vi "日志报警状态存储 (子VI).vi"() -> ()   [LabVIEW 2016, in "斯坦道CODMn.lvlib"]
uses:
  <vilib>/ptbypt/NI_PtbyPt.lvlib
panel:
  out "多列列表框":i32(listbox)
  out "CODMn工作状态":T1(ring)
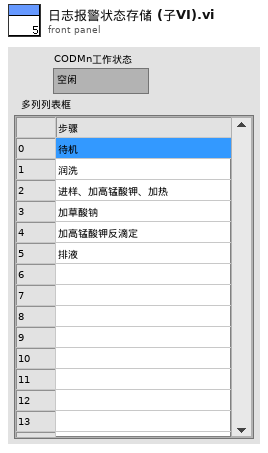
[diagram p1: front panel]
types:
  T1 = enum16{"空闲", "水样测试", "标样核查", "零点核查", "跨度核查", "空白测试", "平行样测试", "质控样", "空白校准", "标样校准", "加标回收"}
  T2 = cluster{"时间标识":timestamp, "设备":string, "日志信息":string, "备注":string}
  T3 = cluster{"时间标识":timestamp, "参数":string, "日志信息":string, "流程参数":string}
  T4 = cluster{"ORP故障":bool, "温控器故障":bool, "加热故障":bool, "高锰酸钾报警":bool, "草酸钠报警":bool, "测量错误":bool, "校零错误":bool, "校标错误":bool, " 进水样超量程":bool, "排液阀故障":bool, "60分钟超时报警":bool, "进样无液体报警":bool}
  T5 = typedef "数据库类型.ctl" = enum16{"Access", "SQLite"}
  T6 = cluster{"测量量程":dbl, "测量精度":dbl, "测量间隔":dbl, "消解温度":dbl, "消解时长":dbl, "空白校准时间":timestamp, "曲线截距":dbl, "曲线斜率":dbl, "测量检出限":dbl, "测量信号值":dbl, "线性相关系数":dbl, "二次多项式系数":dbl, "标样校准时间":timestamp, "稀释倍数":dbl, "三项式系数":dbl, "空白标定系数":dbl, "量程系数":dbl, "F0/ORPA":dbl, "F1/ORPB":dbl, "F2/ORPK":dbl, "F3":dbl, "F4":dbl, "F5":dbl, "F6":dbl, "F7":dbl, "X0/滴定数":dbl, "量程":dbl}
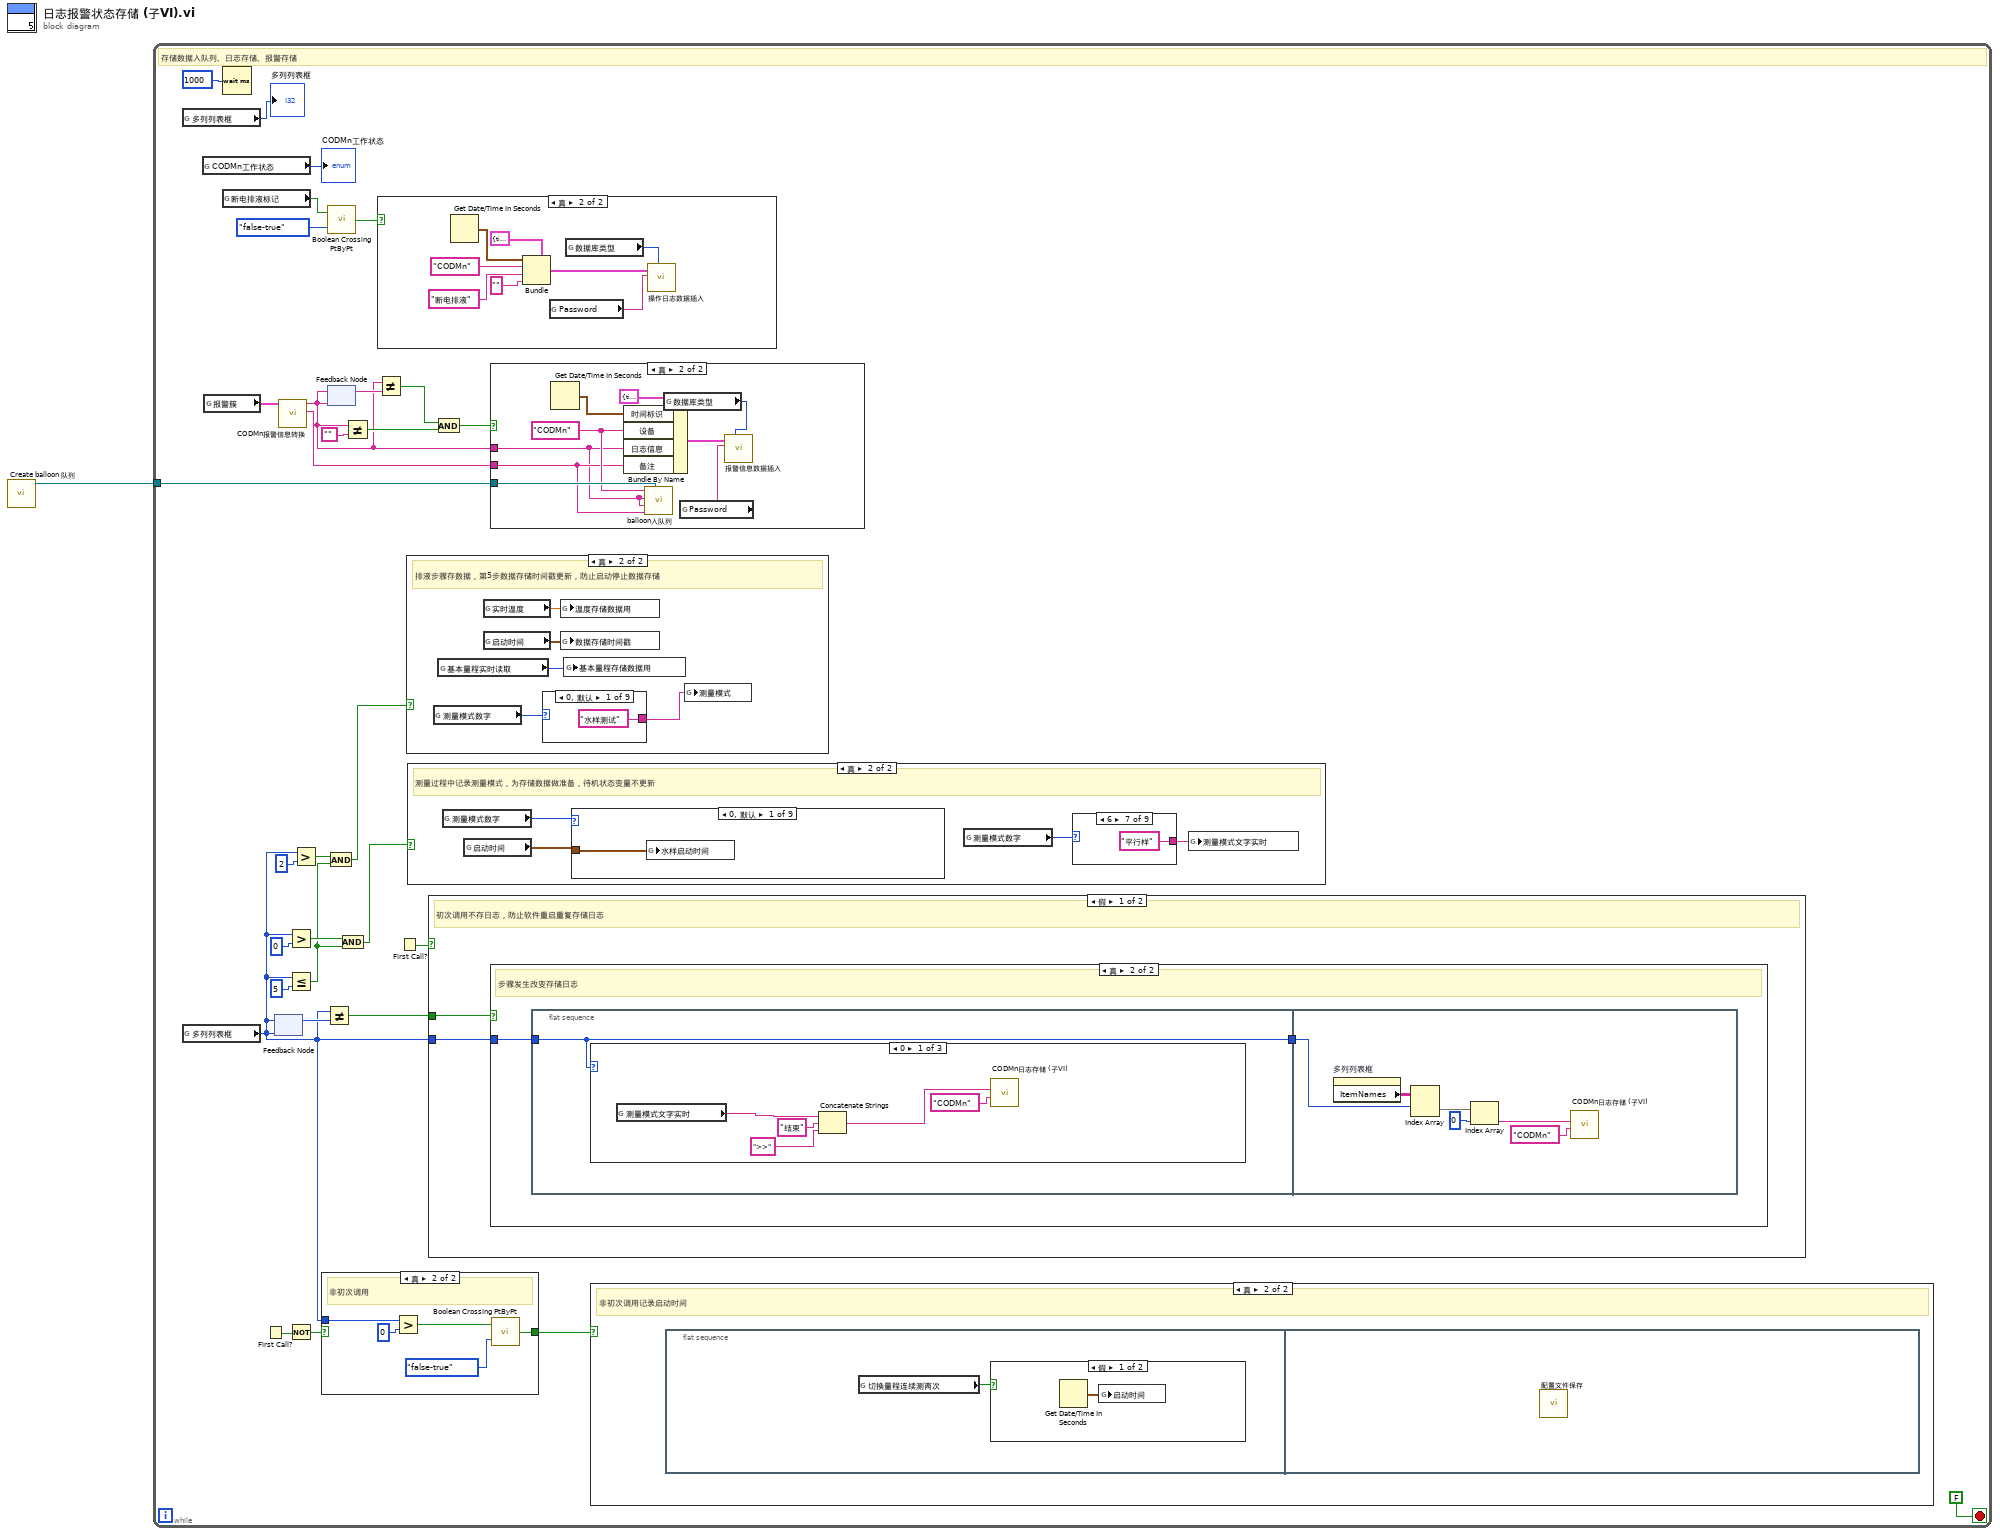
[diagram p0: block diagram]
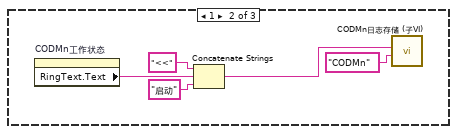
[diagram p3: hidden frame]
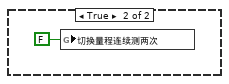
[diagram p10: hidden frame]
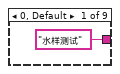
[diagram p12: hidden frame]
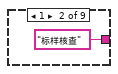
[diagram p13: hidden frame]
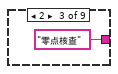
[diagram p14: hidden frame]
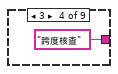
[diagram p15: hidden frame]
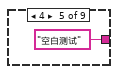
[diagram p16: hidden frame]
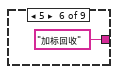
[diagram p17: hidden frame]
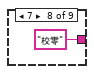
[diagram p18: hidden frame]
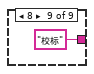
[diagram p19: hidden frame]
diagram:
  n1 = call "Create balloon 队列.vi"() -> ("队列输出"=w1:refnum<queue>)  [unwired: 11 in]
  n2 = while {
    tunnel: w1 -> [w2]
    stop <- FALSE stop-if-true
    # "存储数据入队列、日志存储、报警存储"
    n3 = global read "运行时序全局变量.vi" "多列列表框"() -> (→"多列列表框":i32)
    n4 = global read "运行时序全局变量.vi" "多列列表框"() -> (w6:i32)
    n5 = global read "COD测量模式全局.vi" "CODMn工作状态"() -> (→"CODMn工作状态":T1)
    n6 = global read "COD内部交互全局.vi" "报警簇"() -> (w13:T4)
    n7 = global read "COD内部交互全局.vi" "断电排液标记"() -> (w12:bool)
    n8 = Wait (ms)(milliseconds to wait=u32 1000 ("等待时间（毫秒）")) -> ()  [unwired: 1 out]
    n9 = First Call?() -> (First Call?: T/F=w16:bool)
    n10 = feedback #1(w6) -> (w27:i32)
    n11 = feedback-in #1(w6) -> ()
    n12 = call "CODMn报警信息转换.vi"("报警簇"=w13) -> ("CODMN报警信息备注"=w3:string, "CODMN报警信息"=w17:string)  [unwired: 9 in]
    n13 = Greater?(x=w6, y=u16 0) -> (0:w32:bool)
    n14 = Less Or Equal?(x=w6, y=u16 5) -> (x <= y?=w7:bool)
    n15 = Not(x=w16) -> (.not. x?=w14:bool)
    n16 = Greater?(x=w6, y=u16 2) -> (0:w8:bool)
    n17 = case shown="真" w14 {
      selector: w14 -> [w54 _]
      tunnel: w6 -> [_ w56]
      tunnel: [w54 w55] -> w15
      frame False {
      }
      frame True {
        # "非初次调用"
        n18 = Greater?(x=w56, y=u16 0) -> (0:w59:bool)
        n19 = call <vilib>:"Boolean Crossing PtByPt.vi"("direction"=enum16{"either", "false-true", "true-false"}."false-true", "input"=w59) -> ("crossing"=w55:bool)  [unwired: 1 in]
      }
    }
    n20 = Not Equal?(x=w6, y=w27) -> (x != y?=w28:bool)
    n21 = call <vilib>:"Boolean Crossing PtByPt.vi"("direction"=enum16{"either", "false-true", "true-false"}."false-true", "input"=w12) -> ("crossing"=w23:bool)  [unwired: 1 in]
    n22 = feedback #2(w17) -> (w18:string)
    n23 = feedback-in #2(w17) -> ()
    n24 = And(x=w8, y=w7) -> (x .and. y?=w5:bool)
    n25 = And(x=w32, y=w7) -> (x .and. y?=w4:bool)
    n26 = Not Equal?(x=w17, y="") -> (x != y?=w22:bool)
    n27 = Not Equal?(x=w17, y=w18) -> (x != y?=w19:bool)
    n28 = case shown="真" w23 {
      frame False {
      }
      frame True {
        n29 = Get Date/Time In Seconds() -> (seconds since 1Jan1904=w76:timestamp)
        n30 = Bundle(cluster=T3 {"时间标识"=timestamp(0 s since 1904-01-01), "参数"="", "日志信息"="", "流程参数"=""} ("data in"), "时间标识"=w76, "参数"="CODMn" ("table输入"), "日志信息"="断电排液", "流程参数"="" ("table输入")) -> (w71:T3)
        n31 = global read "CODMn断电保存全局变量.vi" "Password"() -> (w69:string)
        n32 = global read "CODMn断电保存全局变量.vi" "数据库类型"() -> (w70:T5)
        n33 = call "操作日志数据插入.vi"("data"=w71, "Password"=w69, "数据库类型"=w70) -> ()  [unwired: 7 in, 1 out]
      }
    }
    n34 = First Call?() -> (First Call?: T/F=w29:bool)
    n35 = case shown="真" w5 {
      frame False {
      }
      frame True {
        # "排液步骤存数据，第5步数据存储时间戳更新，防止启动停止数据存储"
        n36 = global read "COD内部交互全局.vi" "测量模式数字"() -> (w102:i32)
        n37 = global read "COD内部交互全局.vi" "基本量程实时读取"() -> (w103:enum16{"L", "H", "AUTO"})
        n38 = global read "COD内部交互全局.vi" "实时温度"() -> (w104:dbl)
        n39 = global read "CODMn断电保存全局变量.vi" "启动时间"() -> (w105:timestamp)
        n40 = case shown="0, 默认" w102 {
          tunnel: ["水样测试" ("测量模式") "标样核查" ("测量模式") "零点核查" ("测量模式") "跨度核查" ("测量模式") "空白测试" ("测量模式") "加标回收" ("测量模式") "平行样" ("测量模式") "校零" ("测量模式") "校标" ("测量模式")] -> w101
          frame 0, Default {
          }
          frame 1 {
          }
          frame 2 {
          }
          frame 3 {
          }
          frame 4 {
          }
          frame 5 {
          }
          frame 6 {
          }
          frame 7 {
          }
          frame 8 {
          }
        }
        n41 = global write "COD内部交互全局.vi" "温度存储数据用"(w104) -> ()
        n42 = global write "COD内部交互全局.vi" "数据存储时间戳"(w105) -> ()
        n43 = global write "COD内部交互全局.vi" "基本量程存储数据用"(w103) -> ()
        n44 = global write "CODMn断电保存全局变量.vi" "测量模式"(w101) -> ()
      }
    }
    n45 = case shown="真" w4 {
      frame False {
      }
      frame True {
        # "测量过程中记录测量模式，为存储数据做准备，待机状态变量不更新"
        n46 = global read "COD内部交互全局.vi" "测量模式数字"() -> (w82:i32)
        n47 = global read "CODMn断电保存全局变量.vi" "启动时间"() -> (w83:timestamp)
        n48 = case shown="0, 默认" w82 {
          tunnel: w83 -> [w93 _ _ _ _ w94 _ w95 w98]
          frame 0, Default {
            n49 = global write "COD测量模式全局.vi" "水样启动时间"(w93) -> ()
          }
          frame 1 {
          }
          frame 2 {
          }
          frame 3 {
          }
          frame 4 {
          }
          frame 5 {
            n50 = global write "COD测量模式全局.vi" "加标回收启动时间"(w94) -> ()
          }
          frame 6 {
          }
          frame 7 {
            n51 = global read "CODMn断电保存全局变量.vi" "CODMn仪器参数"() -> (w97:T6)
            n52 = Bundle By Name(cluster=w97, "空白校准时间"=w95) -> (w96:T6)
            n53 = global write "CODMn断电保存全局变量.vi" "CODMn仪器参数"(w96) -> ()
          }
          frame 8 {
            n54 = global read "CODMn断电保存全局变量.vi" "CODMn仪器参数"() -> (w100:T6)
            n55 = Bundle By Name(cluster=w100, "标样校准时间"=w98) -> (w99:T6)
            n56 = global write "CODMn断电保存全局变量.vi" "CODMn仪器参数"(w99) -> ()
          }
        }
        n57 = global read "COD内部交互全局.vi" "测量模式数字"() -> (w80:i32)
        n58 = case shown="6" w80 {
          tunnel: ["水样测试" ("测量模式") "标样核查" ("测量模式") "零点核查" ("测量模式") "跨度核查" ("测量模式") "空白测试" ("测量模式") "加标回收" ("测量模式") "平行样" ("测量模式") "校零" ("测量模式") "校标" ("测量模式")] -> w81
          frame 0, Default {
          }
          frame 1 {
          }
          frame 2 {
          }
          frame 3 {
          }
          frame 4 {
          }
          frame 5 {
          }
          frame 6 {
          }
          frame 7 {
          }
          frame 8 {
          }
        }
        n59 = global write "COD测量模式全局.vi" "测量模式文字实时"(w81) -> ()
      }
    }
    n60 = case shown="假" w29 {
      tunnel: w28 -> [w34 _]
      tunnel: w6 -> [w33 _]
      frame False {
        # "初次调用不存日志，防止软件重启重复存储日志"
        n61 = case shown="真" w34 {
          tunnel: w33 -> [_ w36]
          frame False {
          }
          frame True {
            # "步骤发生改变存储日志"
            n62 = flat-sequence {
              tunnel: w36 -> [w37]
              tunnel: [w37] -> w35
              tunnel: w35 -> [w53]
              frame #0 {
                n63 = case shown="0" w37 {
                  frame 0 {
                    n64 = global read "COD测量模式全局.vi" "测量模式文字实时"() -> (w39:string)
                    n65 = Concatenate Strings(w39, "结束" ("字符串"), ">>") -> (w42:string)
                    n66 = call "CODMn日志存储 (子VI).vi"("参数"="CODMn" ("table输入"), "日志信息"=w42) -> ()  [unwired: 10 in]
                  }
                  frame 1 {
                    n67 = property on="CODMn工作状态" class="Enum (严格)"() -> ("RingText.Text"=w43:string)  [unwired: 2 in, 2 out]
                    n68 = Concatenate Strings("<<", w43, "启动" ("字符串")) -> (w44:string)
                    n69 = call "CODMn日志存储 (子VI).vi"("参数"="CODMn" ("table输入"), "日志信息"=w44) -> ()  [unwired: 10 in]
                  }
                  frame 2, Default {
                  }
                }
              }
              frame #1 {
                n70 = property on="多列列表框" class="MCListbox (严格)"() -> ("ItemNames"=w48:string[][])  [unwired: 2 in, 2 out]
                n71 = Index Array(array=w48, index (row)=w53) -> (element=w51:string[])  [unwired: 1 in]
                n72 = Index Array(array=w51, index=0 ("索引")) -> (element=w49:string)
                n73 = call "CODMn日志存储 (子VI).vi"("参数"="CODMn" ("table输入"), "日志信息"=w49) -> ()  [unwired: 10 in]
              }
            }
          }
        }
      }
      frame True {
      }
    }
    n74 = And(x=w19, y=w22) -> (x .and. y?=w20:bool)
    n75 = case shown="真" w20 {
      tunnel: w17 -> [_ w63]
      tunnel: w3 -> [_ w64]
      tunnel: w2 -> [_ w66]
      frame False {
      }
      frame True {
        w65 = "CODMn" ("设备")
        n76 = Get Date/Time In Seconds() -> (seconds since 1Jan1904=w68:timestamp)
        n77 = Bundle By Name(cluster=T2 {"时间标识"=timestamp(0 s since 1904-01-01), "设备"="", "日志信息"="", "备注"=""} ("data in"), "时间标识"=w68, "设备"=w65, "日志信息"=w63, "备注"=w64) -> (w62:T2)
        n78 = call "balloon入队列.vi"("队列"=w66, "故障详情"=w64, "告警信息"=w63, "故障信息"=w63, "参数名称"=w65) -> ()  [unwired: 6 in, 1 out]
        n79 = global read "CODMn断电保存全局变量.vi" "数据库类型"() -> (w61:T5)
        n80 = global read "CODMn断电保存全局变量.vi" "Password"() -> (w60:string)
        n81 = call "报警信息数据插入.vi"("data"=w62, "Password"=w60, "数据库类型"=w61) -> ()  [unwired: 7 in, 1 out]
      }
    }
    n82 = case shown="真" w15 {
      frame False {
      }
      frame True {
        # "非初次调用记录启动时间"
        n83 = flat-sequence {
          frame #0 {
            n84 = global read "COD内部交互全局.vi" "切换量程连续测两次"() -> (w77:bool)
            n85 = case shown="假" w77 {
              frame False {
                n86 = Get Date/Time In Seconds() -> (seconds since 1Jan1904=w78:timestamp)
                n87 = global write "CODMn断电保存全局变量.vi" "启动时间"(w78) -> ()
              }
              frame True {
                n88 = global write "COD内部交互全局.vi" "切换量程连续测两次"(FALSE ("切换量程连续测两次")) -> ()
              }
            }
          }
          frame #1 {
            n89 = call "配置文件保存.vi"() -> ()  [unwired: 12 in]
          }
        }
      }
    }
  }
